vi "niFpgaSwitchTemplate.vi"(0 "input 1":fxp<+/-,16,16>, 5 "control input":fxp<+/-,16,16>, 7 "input 2":fxp<+/-,16,16>, 12 "threshold":fxp<+/-,16,16>) -> (4 "output":fxp<+/-,16,16>)   [LabVIEW 2017]
doc: "Switches between two input values based on the value of <B>control input</B>. The data type you wire to <B>input 1</B> or <B>input 2</B> determines the <B>output</B> data type."
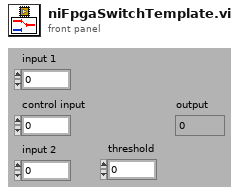
[diagram p1: front panel]
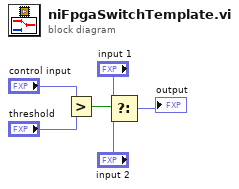
[diagram p0: block diagram]
diagram:
  n1 = Greater?(x="control input", y="threshold") -> (0:w3:bool)
  n2 = Select(t="input 1", s=w3, f="input 2") -> (s? t:f=→"output":fxp<+/-,16,16>)
